vi "GETKTVdll.vi"(8 "error in (no error)":errorcluster, 11 "Inputs":cluster{"icomp":i32, "jcomp":i32}) -> (0 "error out":errorcluster, 3 "Outputs":T1)   [LabVIEW 2015]
doc: "subroutine GETKTVdll(icomp, jcomp, hmodij, fij, hfmix, hfij2, hbinp, hmxrul, hmodij_length, hfmix_length, hfij2_length, hbinp_length, hmxrul_length)\n\nRetrieve mixture model and parameters for a specified binary mixture. \n\nThis subroutine should not be called until after SETUP has been called. The order of icomp and jcomp do not matter, the routine returns the parameters as stored in the hmx.bnc file. To determine if the compositions are backwards, call HMXORDER.\n \nIf callingSETMIX with the same parameters, an error will be returned if the components are backwards.\n\nINPUTS:\nicomp -- component i\njcomp -- component j\n\nOUTPUTS:\nhmodij -- Mixing rule for the binary pair i,j (e.g., KW0, LJ6, or LIN) (character*3)\nfij -- Binary mixture parameters (array of dimension nmxpar; currently\n nmxpar is set to 6); the parameters will vary depending on hmodij;\nhfmix -- File name (character*255) containing parameters for the binary mixture\n model\nhfij2 --description of the binary mixture parameters [character*8\n array of dimension nmxpar]\n for example, for the Lemmon-Jacobsen model (LJ1):\n fij(1) = zeta\n fij(2) = xi\n fij(3) = Fpq\n fij(4) = beta\n fij(5) = gamma\n fij(6) = 'not used'\nhbinp -- Documentation for the binary parameters (character*255)\nhmxrul -- Description of the mixing rule (character*255)\nhmodij_length -- length of variable hmodij (default: 3)\nhfmix_length -- length of variable hfmix (default: 255)\nhfij2_length -- length of variable hfij2 (default: 255)\nhbinp_length -- length of variable hbinp (default: 255)\nhmxrul_length -- length of variable hmxrul (default: 255)"
uses:
  REFPROP.dll
panel:
  # "REFPROP-GETKTVdll.vi"
  # "void  GETKTVdll(int32_t *icomp, int32_t *jcomp, CStr hmodij, double *fij, CStr hfmix, CStr hfij2, CStr hbinp, CStr hmxrul, int32_t hmodij_length, int32_t fmix_length, int32_t hfij2_length, int32_t hbinp_length, int32_t hmrul_length)"
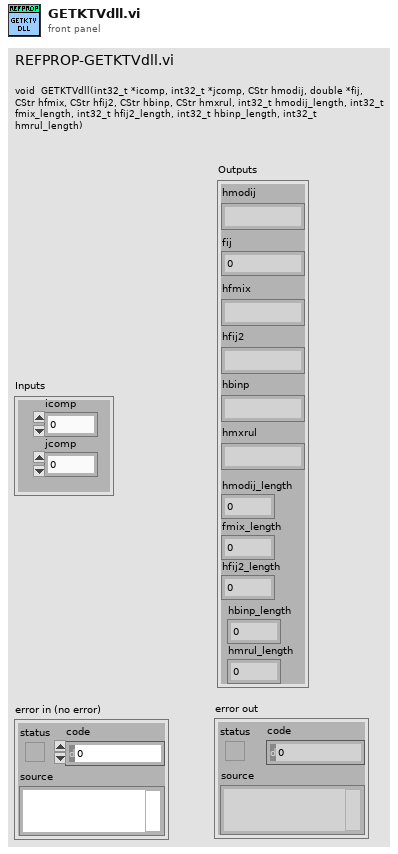
[diagram p1: front panel]
types:
  T1 = cluster{"hmodij":string, "fij":dbl, "hfmix":string, "hfij2":string, "hbinp":string, "hmxrul":string, "hmodij_length":i32, "fmix_length":i32, "hfij2_length":i32, "hbinp_length":i32, "hmrul_length":i32}
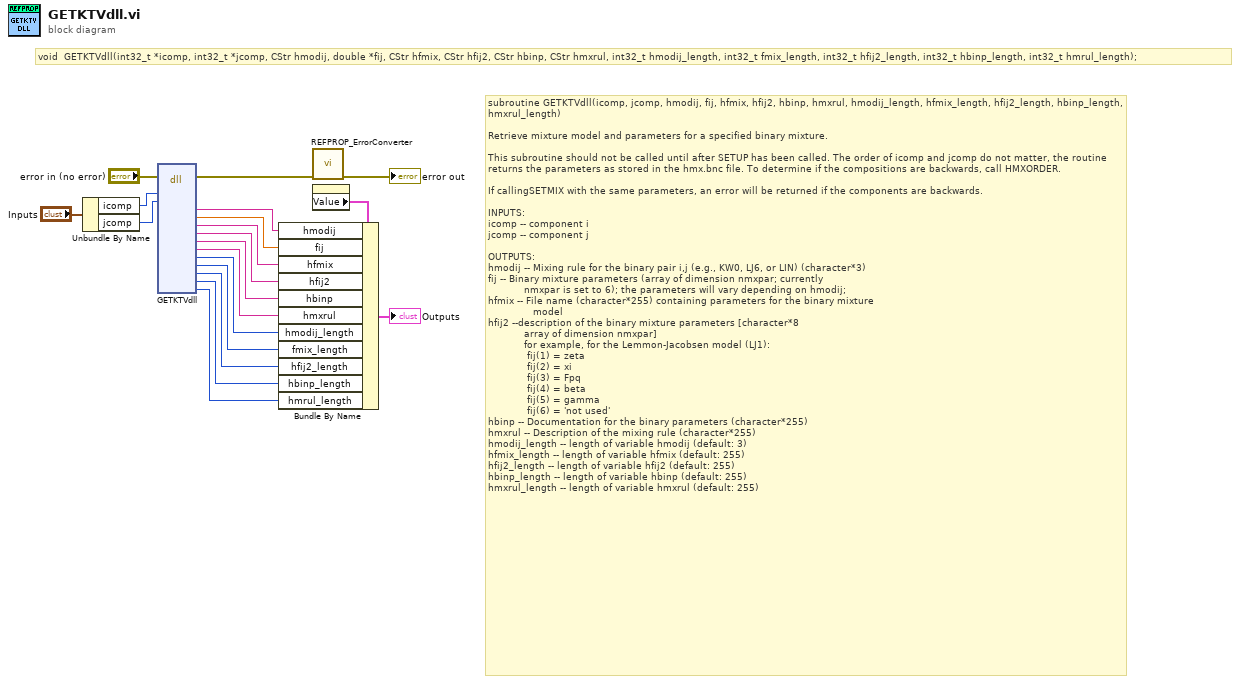
[diagram p0: block diagram]
diagram:
  # "void  GETKTVdll(int32_t *icomp, int32_t *jcomp, CStr hmodij, double *fij, CStr hfmix, CStr hfij2, CStr hbinp, CStr hmxrul, int32_t hmodij_length, int32_t fmix_length, int32_t hfij2_length, int32_t hbinp_length, int32_t hmrul_length);"
  # "subroutine GETKTVdll(icomp, jcomp, hmodij, fij, hfmix, hfij2, hbinp, hmxrul, hmodij_length, hfmix_length, hfij2_length, hbinp_length, hmxrul_length)\n\nRetrieve mixture model and parameters for a specified binary mixture. \n\nThis subroutine should not be called until after SETUP has been called. The order of icomp and jcomp do not matter, the routine returns the parameters as stored in the hmx.bnc file. To determine if the compositions are backwards, call HMXORDER.\n \nIf callingSETMIX with the same parameters, an error will be returned if the components are backwards.\n\nINPUTS:\nicomp -- component i\njcomp -- component j\n\nOUTPUTS:\nhmodij -- Mixing rule for the binary pair i,j (e.g., KW0, LJ6, or LIN) (character*3)\nfij -- Binary mixture parameters (array of dimension nmxpar; currently\n            nmxpar is set to 6); the parameters will vary depending on hmodij;\nhfmix -- File name (character*255) containing parameters for the binary mixture\n               model\nhfij2 --description of the binary mixture parameters [character*8\n            array of dimension nmxpar]\n            for example, for the Lemmon-Jacobsen model (LJ1):\n             fij(1) = zeta\n             fij(2) = xi\n             fij(3) = Fpq\n             fij(4) = beta\n             fij(5) = gamma\n             fij(6) = 'not used'\nhbinp -- Documentation for the binary parameters (character*255)\nhmxrul -- Description of the mixing rule (character*255)\nhmodij_length -- length of variable hmodij (default: 3)\nhfmix_length -- length of variable hfmix (default: 255)\nhfij2_length -- length of variable hfij2 (default: 255)\nhbinp_length -- length of variable hbinp (default: 255)\nhmxrul_length -- length of variable hmxrul (default: 255)"
  n1 = Unbundle By Name("Inputs") -> ("icomp"=w15:i32, "jcomp"=w14:i32)
  n2 = dll-call lib="C:/Users/lauria/Desktop/REFPROP 10 LabVIEW Wrapper BETA/REFPROP/REFPROP.*" fn="GETKTVdll"(error in="error in (no error)", "icomp"=w15, "jcomp"=w14) -> (error out=w19:errorcluster, "hmodij"=w11:string, "fij"=w10:dbl, "hfmix"=w9:string, "hfij2"=w8:string, "hbinp"=w7:string, "hmxrul"=w6:string, "hmodij_length"=w5:i32, "fmix_length"=w4:i32, "hfij2_length"=w3:i32, "hbinp_length"=w2:i32, "hmrul_length"=w1:i32)  [unwired: 16 in, 1 out]
  n3 = call "REFPROP_ErrorConverter.vi"("error in (no error)"=w19) -> ("error out"=→"error out":errorcluster)  [unwired: 10 in]
  n4 = property on="Outputs" class="Clust (strict)"() -> ("Value"=w12:T1)  [unwired: 2 in, 2 out]
  n5 = Bundle By Name(cluster=w12, "hmodij"=w11, "fij"=w10, "hfmix"=w9, "hfij2"=w8, "hbinp"=w7, "hmxrul"=w6, "hmodij_length"=w5, "fmix_length"=w4, "hfij2_length"=w3, "hbinp_length"=w2, "hmrul_length"=w1) -> (→"Outputs":T1)
